vi "LABS5_Ejercicio_noTerminado.vi"() -> ()   [LabVIEW 2012]
panel:
  in  "Fcon":dbl(knob) scale=1.0..20.0
  in  "Offset":dbl
  in  "A":dbl
  out "T":dbl
  in  "Fs":dbl
  in  "Tfinal":dbl
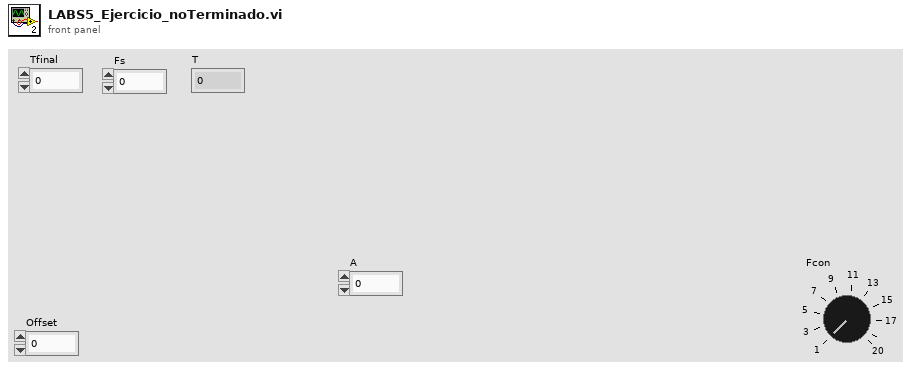
[diagram p1: front panel]
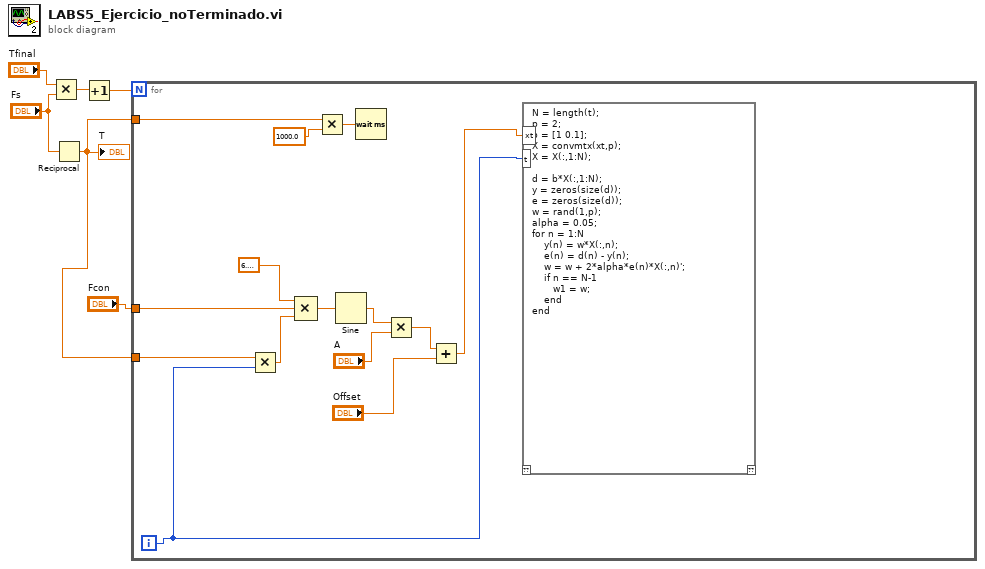
[diagram p0: block diagram]
diagram:
  n1 = Multiply(x="Tfinal", y="Fs") -> (x*y=w5:dbl)
  n2 = Reciprocal(x="Fs") -> (1/x=w1:dbl)
  "T" <- w1
  n3 = Increment(x=w5) -> (x+1=w3:dbl)
  n4 = for {
    N: w3 -> [_]
    tunnel: w1 -> [w18]
    tunnel: "Fcon" -> [w10]
    tunnel: w1 -> [w9]
    i -> [w7]
    n5 = Multiply(x=w9, y=w7) -> (x*y=w16:dbl)
    n6 = Compound Arithmetic op=MULTIPLY(6.283185307179586, w10, w16) -> (w15:dbl)
    n7 = Multiply(x=w18, y=1000.0) -> (x*y=w19:dbl)
    n8 = Sine(x=w15) -> (sin(x)=w14:dbl)
    n9 = Wait (ms)(milliseconds to wait=w19) -> ()  [unwired: 1 out]
    n10 = Multiply(x=w14, y="A") -> (x*y=w12:dbl)
    n11 = Add(x=w12, y="Offset") -> (x+y=w8:dbl)
    n12 = script code="N = length(t);\np = 2;\nb = [1 0.1];\nX = convmtx(xt,p);\nX = X(:,1:N);\n\nd = b*X(:,1:N);\ny = zeros(size(d));\ne = zeros(size(d));\nw = rand(1,p);\nalpha = 0.05;\nfor n = 1:N\n    y(n) = w*X(:,n);\n    e(n) = d(n) - y(n);\n    w = w + 2*alpha*e(n)*X(:,n)';\n    if n == N-1\n       w1 = w; \n    end\nend"("xt"=w8, "t"=w7) -> ()  [unwired: 1 in, 1 out]
  }
